vi "简易流程启动.vi"(8 "Error in":errorcluster caption="Error in (no error)", 9 "简易流程":u16(ring), 10 "参数Id":u16, 11 "MB session in":refnum<class "MB_Master.lvclass">) -> (0 "error out":errorcluster, 3 "MB session out":refnum<class "MB_Master.lvclass">)   [LabVIEW 2016, in "斯坦道通用流路CODmn.lvlib"]
uses:
  <vilib>/Plasmionique/MB Master/MB_Master/MB_Master.lvclass
  <vilib>/Plasmionique/MB Master/MB Master.lvlib
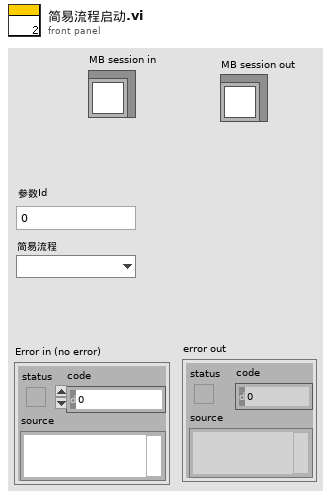
[diagram p1: front panel]
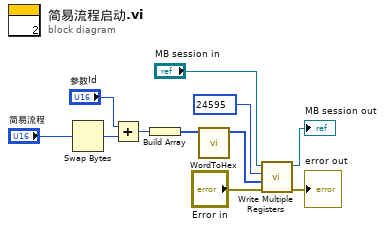
[diagram p0: block diagram]
diagram:
  n1 = Swap Bytes(anything="简易流程") -> (byte swapped=w4:u16)
  n2 = Add(x="参数Id", y=w4) -> (x+y=w2:u16)
  n3 = Build Array(w2) -> (w1:u16[])
  n4 = call "WordToHex.vi"("WORD"=w1) -> ("数组"=w6:u16[])  [unwired: 10 in]
  n5 = call <vilib>:"Write Multiple Registers.vi"("error in (no error)"="Error in", "values"=w6, "starting address"=u16 24595, "MB session in"="MB session in") -> ("error out"=→"error out":errorcluster, "MB session out"=→"MB session out":refnum<class "MB_Master.lvclass">)  [unwired: 6 in]
